vi "Pre Launch Init.vi"(11 "UI Actor in":refnum<class "UI Actor.lvclass">) -> (0 "error out":errorcluster, 3 "UI Actor out":refnum<class "UI Actor.lvclass">)   [LabVIEW 2024, in "UI Actor.lvlib" / "UI Actor.lvclass"]
doc: "Initializes the panel actor. Creates the Panel Helper.\n\n----\nPlease see the following web address for additional documentation and tutorial information:\nhttp://www.mooregoodideas.com/mgi-panel-manager/\n\nAuthor: Derek Trepanier\n\nCopyright (c) 2018, Moore Good Ideas, Inc.\n\nAll rights reserved.\n\nRedistribution and use in source and binary forms, with or without modification, are permitted provided that the following conditions are met:\n\n * Redistributions of source code must retain the above copyright notice, this list of conditions and the following disclaimer.\n * Redistributions in binary form must reproduce the above copyright notice, this list of conditions and the following disclaimer in the documentation and/or other materials provided with the distribution.\n * Neither the name of Moore Good Ideas, Inc. nor the names of its contributors may be used to endorse or promote products derived from this software without specific prior written permission.\n\nTHIS SOFTWARE IS PROVIDED BY THE COPYRIGHT HOLDERS AND CONTRIBUTORS \"AS IS\" AND ANY EXPRESS OR IMPLIED WARRANTIES, INCLUDING, BUT NOT LIMITED TO, THE IMPLIED WARRANTIES OF MERCHANTABILITY AND FITNESS FOR A PARTICULAR PURPOSE ARE DISCLAIMED. IN NO EVENT SHALL THE COPYRIGHT OWNER OR CONTRIBUTORS BE LIABLE FOR ANY DIRECT, INDIRECT, INCIDENTAL, SPECIAL, EXEMPLARY, OR CONSEQUENTIAL DAMAGES (INCLUDING, BUT NOT LIMITED TO, PROCUREMENT OF SUBSTITUTE GOODS OR SERVICES; LOSS OF USE, DATA, OR PROFITS; OR BUSINESS INTERRUPTION) HOWEVER CAUSED AND ON ANY THEORY OF LIABILITY, WHETHER IN CONTRACT, STRICT LIABILITY, OR TORT (INCLUDING NEGLIGENCE OR OTHERWISE) ARISING IN ANY WAY OUT OF THE USE OF THIS SOFTWARE, EVEN IF ADVISED OF THE POSSIBILITY OF SUCH DAMAGE."
uses:
  UI Actor.lvclass
  UI Actor.lvclass/UI Actor.ctl
  <vilib>/MGI/Panel Manager/Panel Actor/Panel Actor/Panel Actor.lvclass
  Controls/Supported Baudrates.ctl
  UI Actor.lvlib
  Controls/Device Info.ctl
  Controls/File Info.ctl
  Controls/Device Settings.ctl
  Core/Object Type.ctl
  Core/Electronic Datasheet.lvlib
  Core/Access SDO.ctl
  Core/Access PDO.ctl
  Core/Access SRDO.ctl
  Controls/TX Communication Parameter.ctl
  Controls/RX Communication Parameter.ctl
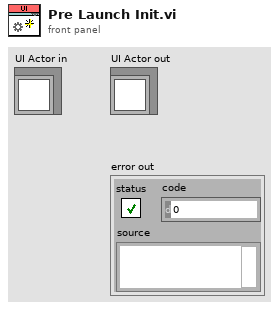
[diagram p1: front panel]
types:
  T1 = typedef "UI Actor.lvlib/UI Actor.lvclass/RX Communication Parameter.ctl" = cluster{"Communication":u16, "Mapping":u16, "COB":u32, "Transm. Type":u8, "Inhibit":u16, "Event Timer":u16, "Sync Start":u8}
  T2 = typedef "UI Actor.lvlib/UI Actor.lvclass/TX Communication Parameter.ctl" = cluster{"Communication":u16, "Mapping":u16, "COB":u32, "Type":u8, "Inhibit":u16, "Event Timer":u16, "Sync Start":u8}
  T3 = typedef "Electronic Datasheet.lvlib/Object Type.ctl" = u8
  T4 = typedef "Electronic Datasheet.lvlib/Access SDO.ctl" = enum16{"read only", "write only", "read/write", "read/write on process input", "read/write on process output", "constant value", "no", "UNKNOWN"}
  T5 = typedef "Electronic Datasheet.lvlib/Access PDO.ctl" = enum16{"no", "TPDO", "RPDO", "TPDO & RPDO"}
  T6 = typedef "Electronic Datasheet.lvlib/Access SRDO.ctl" = enum16{"no", "tx", "rx", "trx"}
  T7 = cluster{"ParameterName":string, "Description":string, "ObjectType":T3, "DataType":u16, "DefaultValue":string, "Denotation":string, "HighLimit":string, "LowLimit":string, "Access SDO":T4, "Access PDO":T5, "Access SRDO":T6, "Actual Value":string}
  T8 = typedef "UI Actor.lvlib/Device Settings.ctl" = cluster{"SimpleBootUpSlave":bool, "SimpleBootUpMaster":bool}
  T9 = typedef "UI Actor.lvlib/File Info.ctl" = cluster{"FileVersion":u8, "FileRevision":u8, "EDSVersion":string, "Description":string, "CreationDate":string, "CreationTime":string, "CreatedBy":string, "ModificationDate":string, "ModificationTime":string, "ModifiedBy":string}
  T10 = typedef "UI Actor.lvlib/Device Info.ctl" = cluster{"ProductName":string, "ProductNumber":u32, "VendorName":string, "VendorNumber":u32}
  T11 = typedef "UI Actor.lvlib/Supported Baudrates.ctl" = cluster{"BaudRate_10":bool, "BaudRate_20":bool, "BaudRate_50":bool, "BaudRate_125":bool, "BaudRate_250":bool, "BaudRate_500":bool, "BaudRate_800":bool, "BaudRate_1000":bool, "BaudRate_auto":bool}
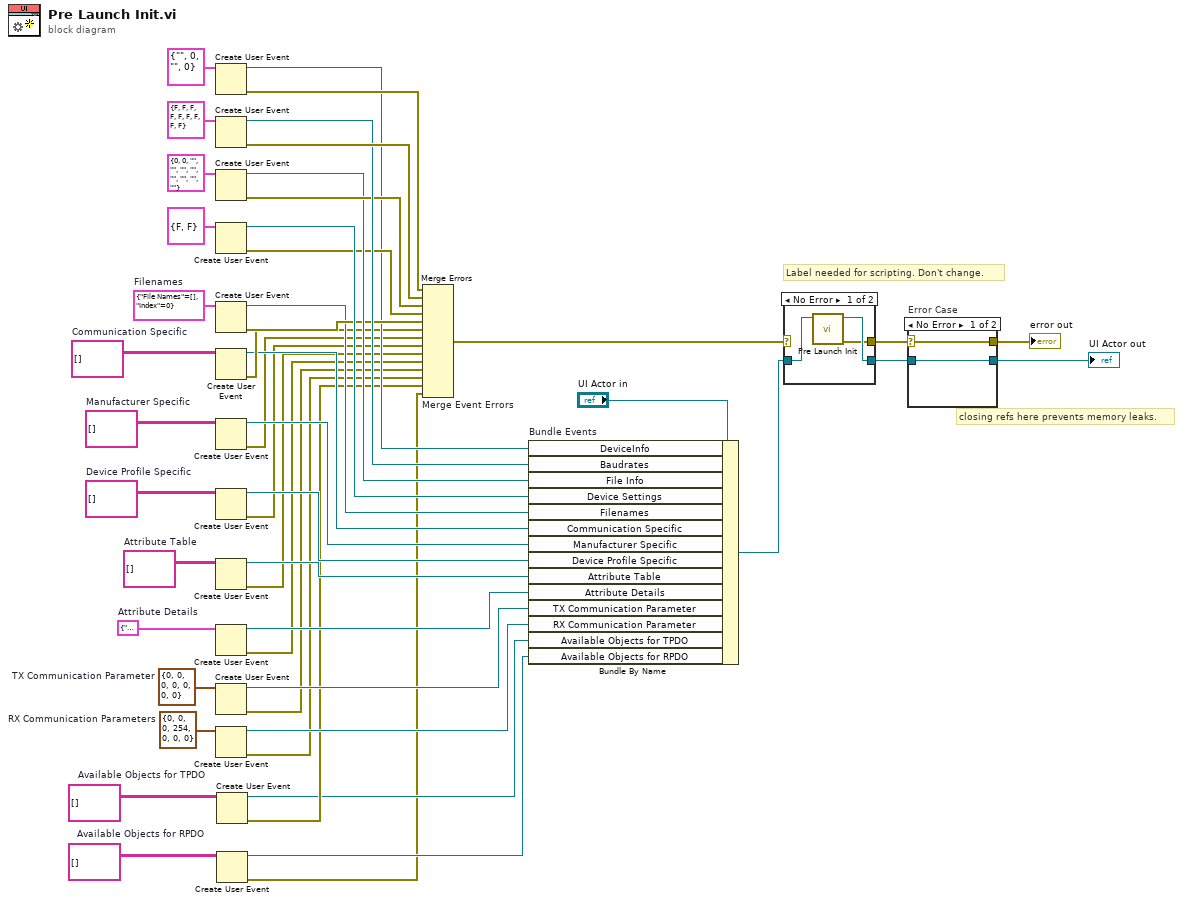
[diagram p0: block diagram]
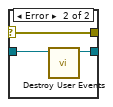
[diagram p3: hidden frame]
diagram:
  w3 = string[][] []  # Available Objects for RPDO
  w6 = string[][] []  # Available Objects for TPDO
  w7 = T1 {"Communication"=0, "Mapping"=0, "COB"=0, "Transm. Type"=254, "Inhibit"=0, "Event Timer"=0, "Sync Start"=0}  # RX Communication Parameters
  w8 = T2 {"Communication"=0, "Mapping"=0, "COB"=0, "Type"=0, "Inhibit"=0, "Event Timer"=0, "Sync Start"=0}  # TX Communication Parameter
  w15 = T7 {"ParameterName"="", "Description"="", "ObjectType"=0, "DataType"=0, "DefaultValue"="", "Denotation"="", "HighLimit"="", "LowLimit"="", "Access SDO"=enum."read only", "Access PDO"=enum."no", "Access SRDO"=enum."no", "Actual Value"=""}  # Attribute Details
  w18 = string[][] []  # Attribute Table
  w23 = string[][] []  # Device Profile Specific
  w24 = string[][] []  # Manufacturer Specific
  w26 = string[][] []  # Communication Specific
  w30 = cluster{"File Names":string[], "Index":i32} {"File Names"=[], "Index"=0}  # Filenames
  # "closing refs here prevents memory leaks."
  # "Label needed for scripting. Don't change."
  n1 = Create User Event(user event datatype=T10 {"ProductName"="", "ProductNumber"=0, "VendorName"="", "VendorNumber"=0} ("DeviceInfo")) -> (user event=w28:refnum<user-event>, error out=w43:errorcluster)  [unwired: 1 in]
  n2 = Create User Event(user event datatype=T11 {"BaudRate_10"=FALSE, "BaudRate_20"=FALSE, "BaudRate_50"=FALSE, "BaudRate_125"=FALSE, "BaudRate_250"=FALSE, "BaudRate_500"=FALSE, "BaudRate_800"=FALSE, "BaudRate_1000"=FALSE, "BaudRate_auto"=FALSE} ("Baudrates")) -> (user event=w38:refnum<user-event>, error out=w39:errorcluster)  [unwired: 1 in]
  n3 = Create User Event(user event datatype=T9 {"FileVersion"=0, "FileRevision"=0, "EDSVersion"="", "Description"="", "CreationDate"="", "CreationTime"="", "CreatedBy"="", "ModificationDate"="", "ModificationTime"="", "ModifiedBy"=""} ("EDS File Info")) -> (user event=w35:refnum<user-event>, error out=w36:errorcluster)  [unwired: 1 in]
  n4 = Create User Event(user event datatype=T8 {"SimpleBootUpSlave"=FALSE, "SimpleBootUpMaster"=FALSE} ("Device Settings")) -> (user event=w33:refnum<user-event>, error out=w32:errorcluster)  [unwired: 1 in]
  n5 = Create User Event(user event datatype=w30) -> (user event=w29:refnum<user-event>, error out=w31:errorcluster)  [unwired: 1 in]
  n6 = Create User Event(user event datatype=w26) -> (user event=w25:refnum<user-event>, error out=w27:errorcluster)  [unwired: 1 in]
  n7 = Create User Event(user event datatype=w24) -> (user event=w22:refnum<user-event>, error out=w20:errorcluster)  [unwired: 1 in]
  n8 = Create User Event(user event datatype=w23) -> (user event=w21:refnum<user-event>, error out=w19:errorcluster)  [unwired: 1 in]
  n9 = Create User Event(user event datatype=w18) -> (user event=w17:refnum<user-event>, error out=w16:errorcluster)  [unwired: 1 in]
  n10 = Create User Event(user event datatype=w15) -> (user event=w14:refnum<user-event>, error out=w13:errorcluster)  [unwired: 1 in]
  n11 = Create User Event(user event datatype=w8) -> (user event=w12:refnum<user-event>, error out=w11:errorcluster)  [unwired: 1 in]
  n12 = Create User Event(user event datatype=w7) -> (user event=w10:refnum<user-event>, error out=w9:errorcluster)  [unwired: 1 in]
  n13 = Create User Event(user event datatype=w6) -> (user event=w4:refnum<user-event>, error out=w5:errorcluster)  [unwired: 1 in]
  n14 = Create User Event(user event datatype=w3) -> (user event=w2:refnum<user-event>, error out=w1:errorcluster)  [unwired: 1 in]
  n15 = Merge Errors "Merge Event Errors"(w43, w39, w36, w32, w31, w27, w20, w19, w16, w13, w11, w9, w5, w1) -> (w42:errorcluster)
  n16 = Bundle By Name "Bundle Events"(cluster="UI Actor in", "DeviceInfo"=w28, "Baudrates"=w38, "File Info"=w35, "Device Settings"=w33, "Filenames"=w29, "Communication Specific"=w25, "Manufacturer Specific"=w22, "Device Profile Specific"=w21, "Attribute Table"=w17, "Attribute Details"=w14, "TX Communication Parameter"=w12, "RX Communication Parameter"=w10, "Available Objects for TPDO"=w4, "Available Objects for RPDO"=w2) -> (w44:refnum<class "UI Actor.lvclass">)
  n17 = case shown="No Error" w42 {
    selector: w42 -> [_ w53]
    tunnel: w44 -> [w52 w54]
    tunnel: [w51 w54] -> w49
    tunnel: [w50 w53] -> w47
    frame No Error {
      n18 = call-parent "Pre Launch Init.vi"("Panel Actor in"=w52) -> ("error out"=w50:errorcluster, "Panel Actor out"=w51:refnum<class "UI Actor.lvclass">)  [unwired: 9 in]
    }
    frame Error {
    }
  }
  n19 = case "Error Case" shown="No Error" w47 {
    selector: w47 -> [w55 w59]
    tunnel: w49 -> [w56 w58]
    tunnel: [w56 w57] -> w48
    tunnel: [w55 w59] -> w46
    frame No Error {
    }
    frame Error {
      n20 = call "Destroy User Events.vi"("UI Actor in"=w58) -> ("UI Actor out"=w57:refnum<class "UI Actor.lvclass">)  [unwired: 10 in]
    }
  }
  "error out" <- w46
  "UI Actor out" <- w48
